vi "GLDL Main.vi"() -> ()   [LabVIEW 2018]
doc: "This template is for the Queued Message Handler design pattern.\n\nThe Event Handling Loop generates messages based on user interface actions.\n\nThe Message Handling Loop processes messages generated by the Event Handling Loop, or by other messages. The messages are string values, so new messages can be added easily to the Message Cases case structure in the Message Handling Loop. Each message cluster can also provide an optional value for Message Data, which is a variant that can be converted to whatever message-specific data is required."
uses:
  controls/GLDL UI Data.ctl
  support/Message Queue/GLDL Message Queue.lvlib
  support/User Event - Stop/GLDL User Event - Stop.lvlib
  support/Message Queue/Enqueue Message (Single).vi
  support/Error Handling/GLDL Error Handling.lvlib
  <vilib>/ErrorRing/Error Ring.xnode
  <vilib>/Utility/error.llb/Error Cluster From Error Code.vi
  support/Message Queue/Message Cluster.ctl
  support/Message Queue/All Message Queues.ctl
  Great Lakes Downloads/support/Message Queue/Enqueue Message (Single).vi
  controls/Connected Indicator.ctl
  controls/Processing Loop State.ctl
  controls/Output Indicator.ctl
  controls/Save Path Control.ctl
  controls/COM Port Control.ctl
  controls/Date Control.ctl
  controls/Disconnect Control.ctl
  controls/Clear Control.ctl
  controls/Exit Control.ctl
  controls/Download Control.ctl
  controls/Station ID Indicator.ctl
  controls/Reboot Control.ctl
  controls/IP Phone Number Control.ctl
panel:
  in  "End Time":T1=timestamp(3579694921.225491 s since 1904-01-01) format="%<%m/%d/%Y %H:%M:%S>T"
  in  "Password":string="akl"
  in  "Username":string="super"
  in  "REBOOT":T2
  out "Station ID":T3
  in  "Start Time":T1=timestamp(3579694921.225491 s since 1904-01-01) format="%<%m/%d/%Y %H:%M:%S>T"
  out "Connected?":T4
  in  "Modem COM Port":T5="COM1"
  in  "Clear Indicator":T6
  in  "IP or Phone Number":T7="9,17578424450"
  in  "Save Path":T8
  out "Output":T9
  in  "Download Data":T10
  in  "Connect to Station":T11
  in  "Exit":T12
  # "9,,,17578424450"
  # "9,14197981041,,,#33,,#33,,#33,,#33"
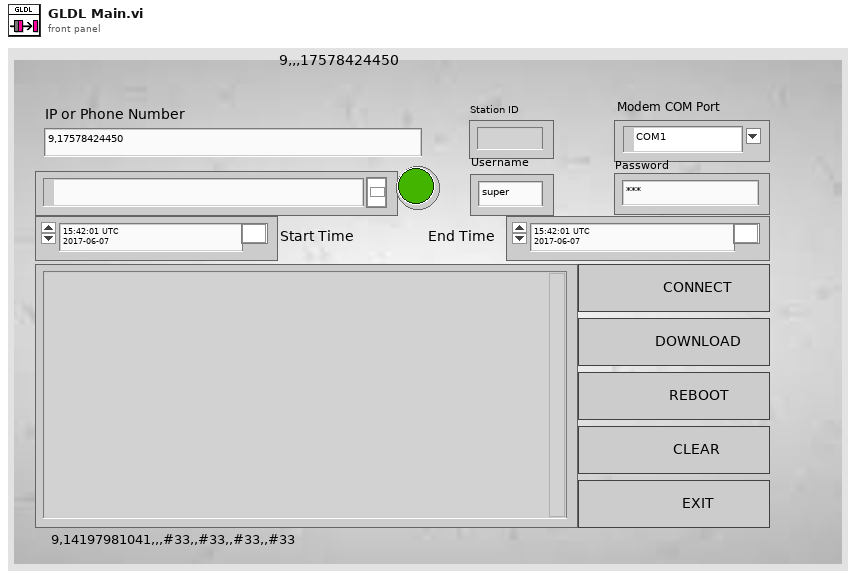
[diagram p1: front panel]
types:
  T1 = typedef "Date Control.ctl" = timestamp
  T2 = typedef "Reboot Control.ctl" = bool
  T3 = typedef "Station ID Indicator.ctl" = string
  T4 = typedef "Connected Indicator.ctl" = bool
  T5 = typedef "COM Port Control.ctl" = refnum<visa-resource-name>
  T6 = typedef "Clear Control.ctl" = bool
  T7 = typedef "IP Phone Number Control.ctl" = string
  T8 = typedef "Save Path Control.ctl" = path
  T9 = typedef "Output Indicator.ctl" = string
  T10 = typedef "Download Control.ctl" = bool
  T11 = typedef "Disconnect Control.ctl" = bool
  T12 = typedef "Exit Control.ctl" = bool
  T13 = typedef "GLDL UI Data.ctl" = cluster{"Data Display":string, "FP Control Refs":cluster{"Connect to Station Ref":refnum<vi>, "Download Ref":refnum<vi>, "Exit Button Ref":refnum<vi>, "Start Date Refnum":refnum<vi>, "End Date Refnum":refnum<vi>, "Path":refnum<vi>, "COM Port":refnum<visa-resource-name>, "IP or Phone Ref":refnum<vi>, "TCPIP ID":refnum<k5>, "Reboot Refnum":refnum<vi>, "Datafile Refnum":refnum<file>}, "FP Indicator Refs":cluster{"Connected Refnum":refnum<vi>, "Data Display Ref":refnum<vi>, "Station ID Ref":refnum<vi>}, "User Events":cluster{"Stop":refnum<user-event>, "Update Display":refnum<user-event>}, "Message Queues":T14, "IS IP?":bool, "Downloading?":bool, "DCP Version":enum16{"XPert", "XPert2"}, "Processing Loop State":T15, "Username":refnum<vi>, "Password":refnum<vi>}
  T14 = typedef "GLDL Message Queue.lvlib/All Message Queues.ctl" = cluster{"UI":refnum<queue>, "ACQUISITION":refnum<queue>, "PROCESSING":refnum<queue>, "LOGGING":refnum<queue>}
  T15 = typedef "Processing Loop State.ctl" = enum16{"Get Station  ID", "Change Directory SD Card", "Change Directory Storage Card", "Downloading", "Idle in DL Directory"}
  T16 = cluster{"Stop":refnum<user-event>, "Update Display":refnum<user-event>}
  T17 = enum16{"Standard", "Buffered", "CRLF", "Immediate"}
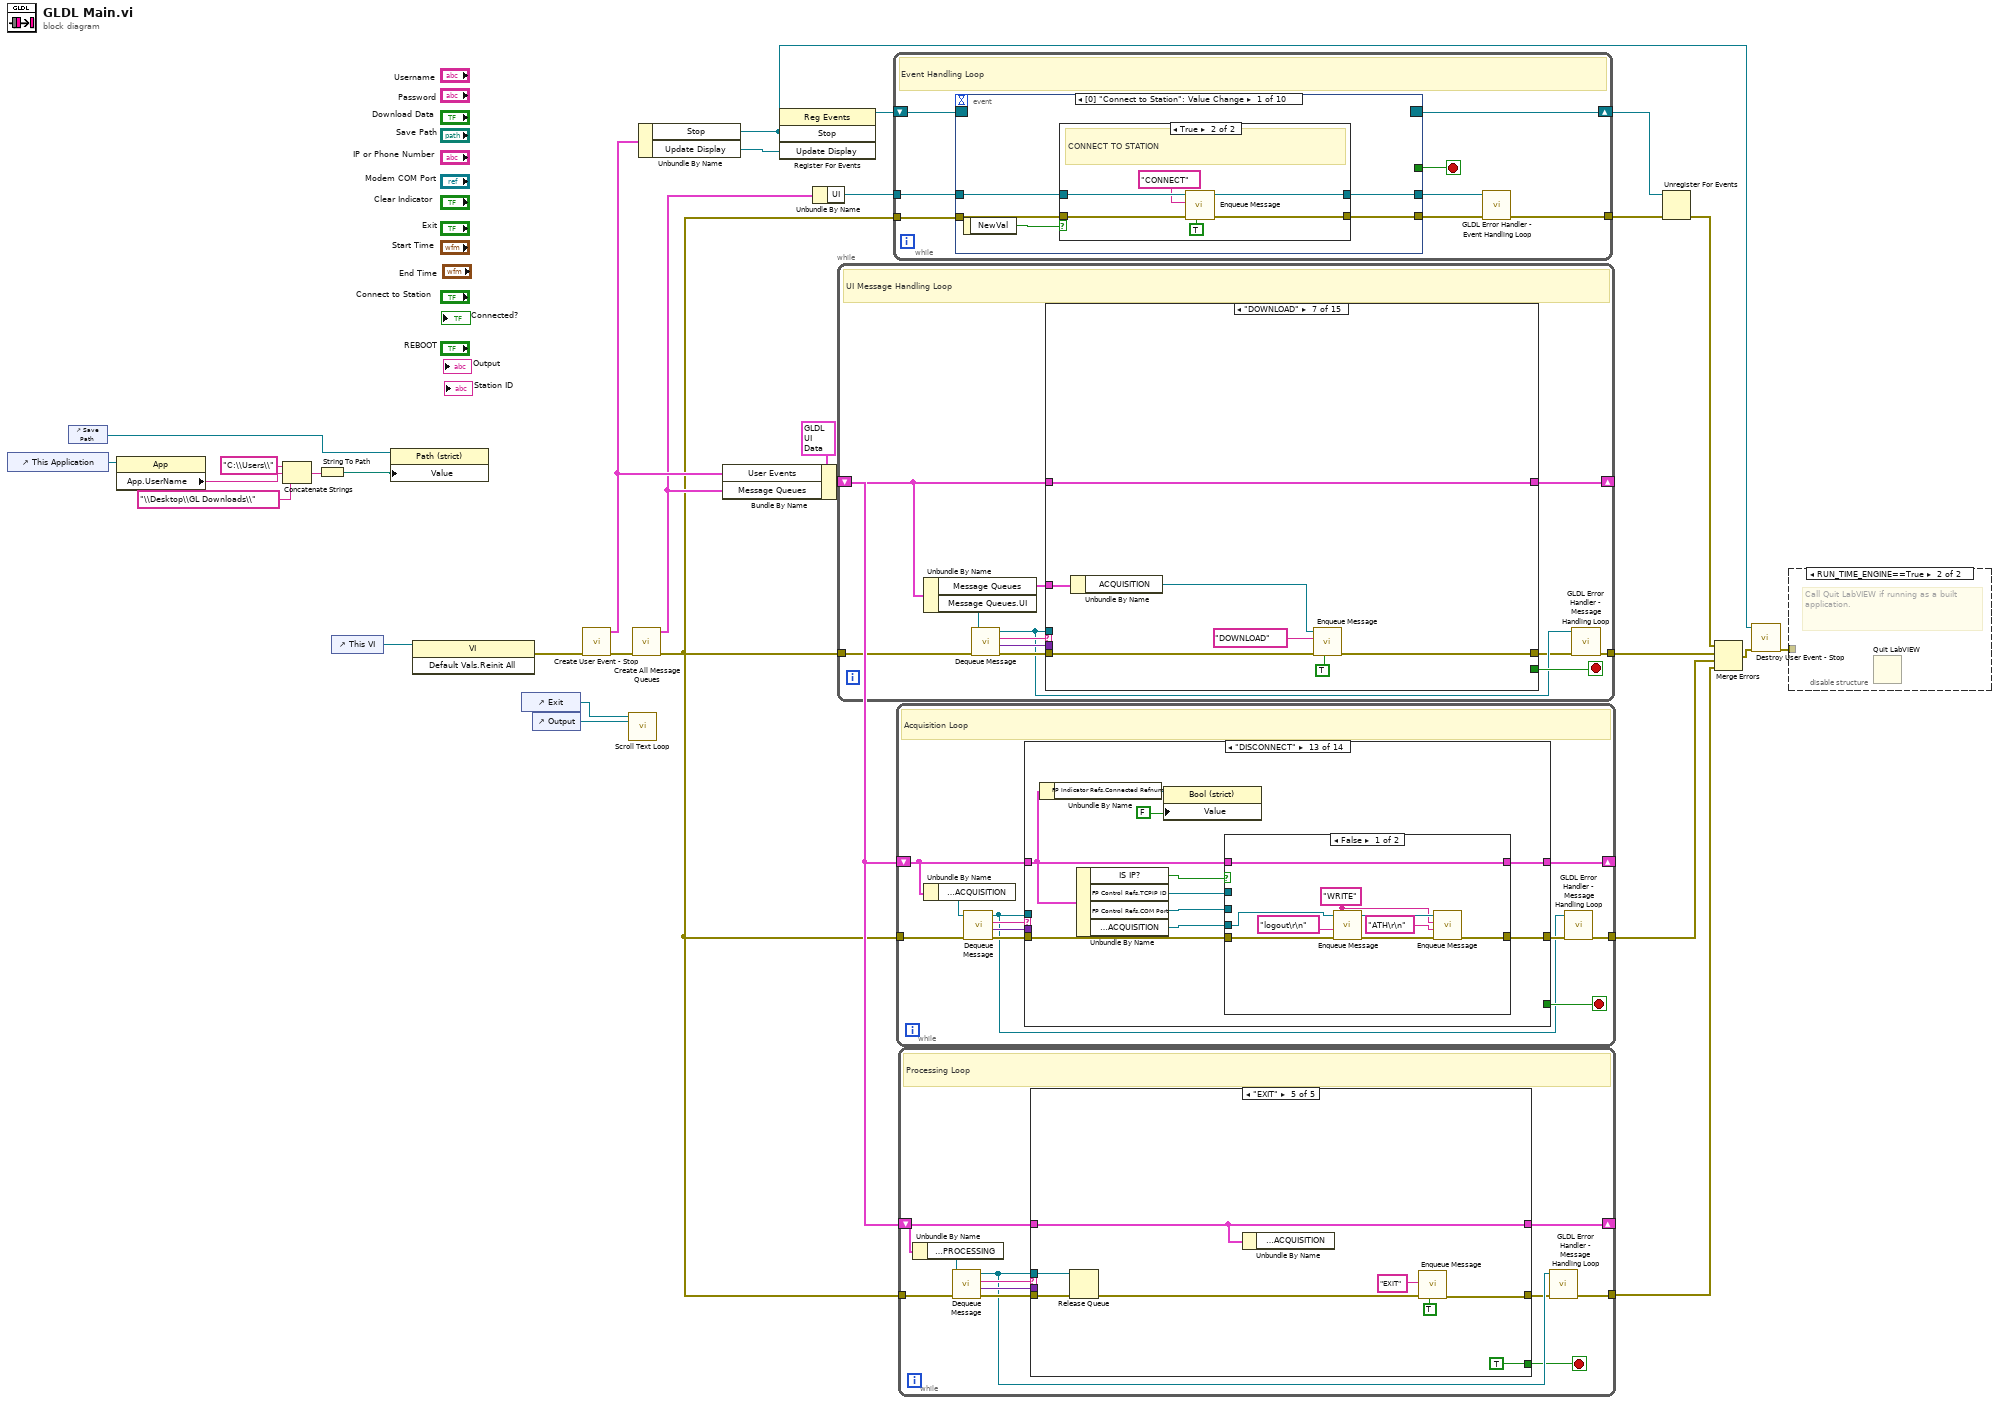
[diagram p0: block diagram]
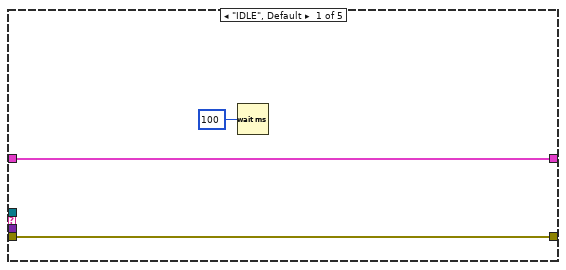
[diagram p2: hidden frame]
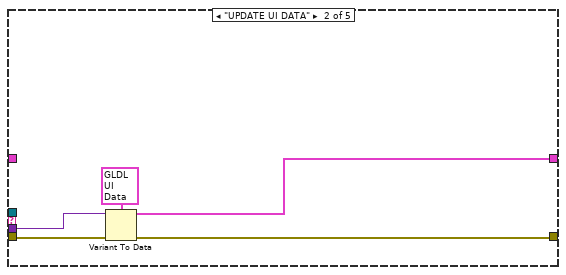
[diagram p3: hidden frame]
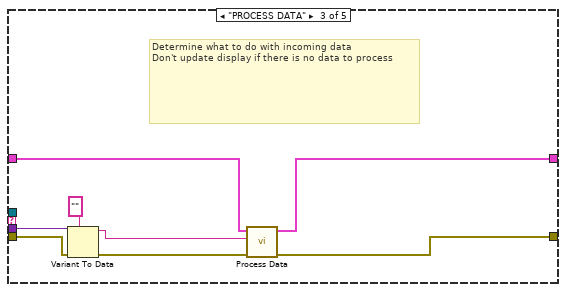
[diagram p4: hidden frame]
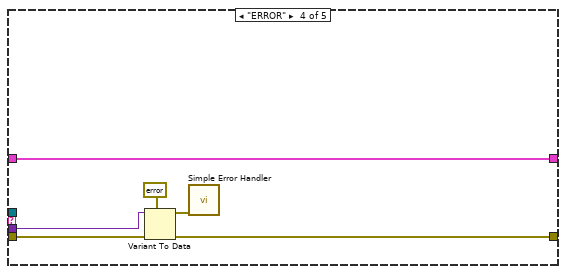
[diagram p5: hidden frame]
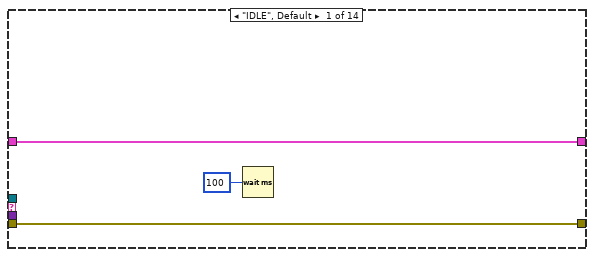
[diagram p6: hidden frame]
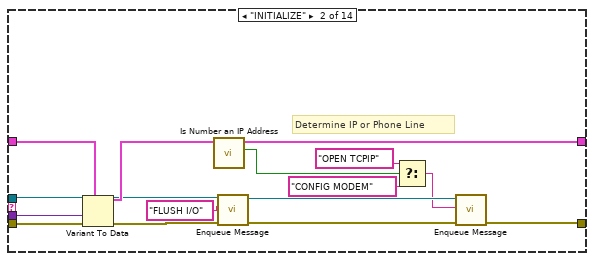
[diagram p7: hidden frame]
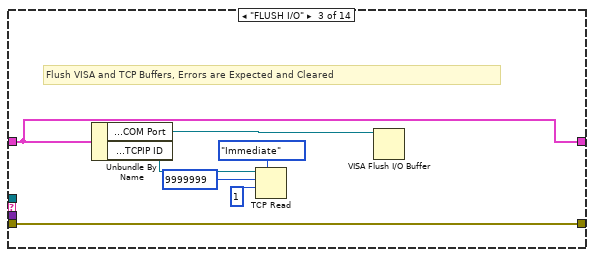
[diagram p8: hidden frame]
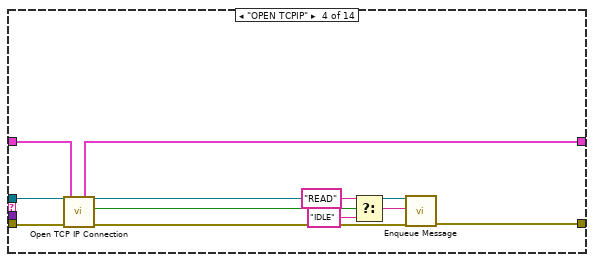
[diagram p9: hidden frame]
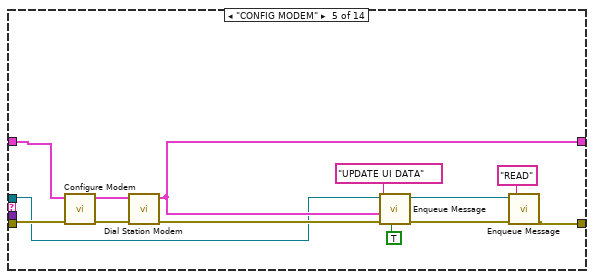
[diagram p10: hidden frame]
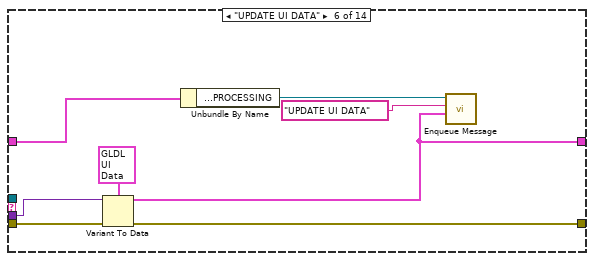
[diagram p11: hidden frame]
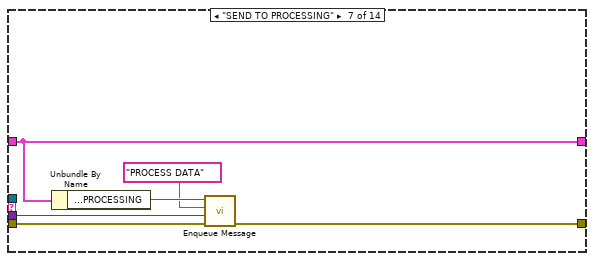
[diagram p12: hidden frame]
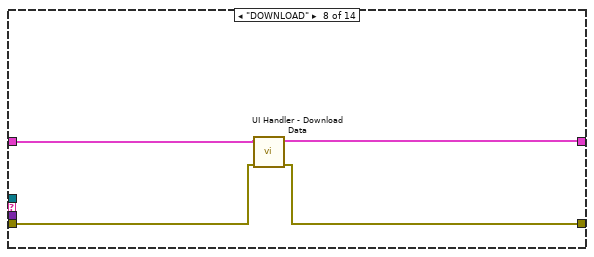
[diagram p13: hidden frame]
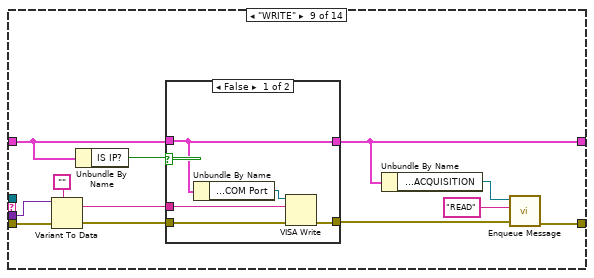
[diagram p14: hidden frame]
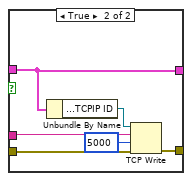
[diagram p15: hidden frame]
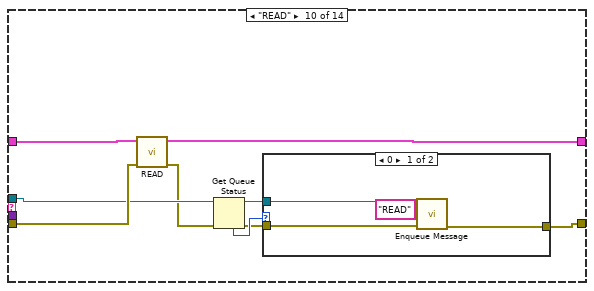
[diagram p16: hidden frame]
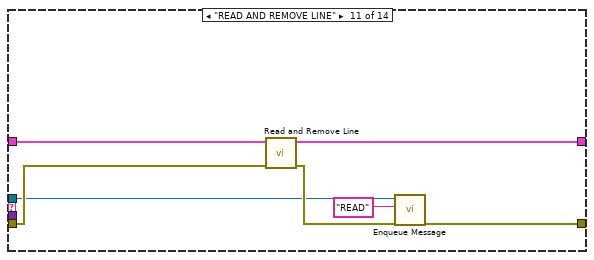
[diagram p18: hidden frame]
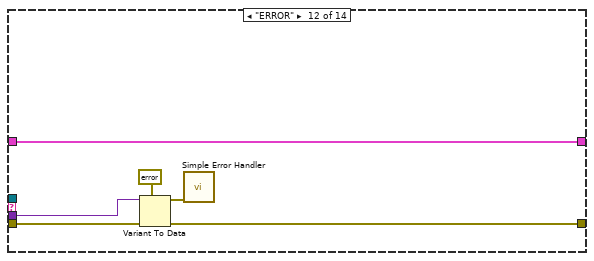
[diagram p19: hidden frame]
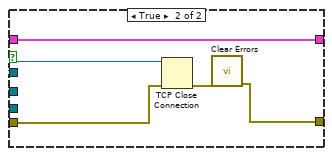
[diagram p20: hidden frame]
diagram:
  n1 = control-ref of="This Application"() -> (w9:refnum<vi>)
  n2 = control-ref of="Save Path"() -> (w3:refnum<vi>)
  n3 = property class="App"(reference=w9) -> ("App.UserName"=w7:string)  [unwired: 1 in, 2 out]
  n4 = Concatenate Strings("C:\\Users\\" ("string"), w7, "\\Desktop\\GL Downloads\\" ("string")) -> (w5:string)
  n5 = String To Path(string=w5) -> (path=w4:path)
  n6 = control-ref of="This VI"() -> (w16:refnum<vi>)
  n7 = property on="Property Node" class="Path (strict)"(reference=w3, "Value"=w4) -> ()  [unwired: 1 in, 2 out]
  n8 = invoke class="VI" method="Default Vals.Reinit All"(reference=w16) -> (error out=w15:errorcluster)  [unwired: 2 in, 2 out]
  n9 = control-ref of="Exit"() -> (w1:refnum<vi>)
  n10 = control-ref of="Output"() -> (w2:refnum<vi>)
  n11 = call "Create User Event - Stop.vi"("error in (no error)"=w15) -> ("error out"=w27:errorcluster, "User Events"=w17:T16)  [unwired: 9 in]
  n12 = call "Scroll Text Loop.vi"("Output Ref"=w2, "Exit Ref"=w1) -> ()  [unwired: 10 in]
  n13 = call "Create All Message Queues.vi"("error in (no error)"=w27) -> ("error out"=w10:errorcluster, "Message Queues out"=w13:T14)  [unwired: 9 in]
  n14 = Unbundle By Name(w17) -> ("Stop"=w20:refnum<user-event>, "Update Display"=w19:refnum<user-event>)
  n15 = Bundle By Name(cluster=T13 {"Data Display"="", "FP Control Refs"={"Connect to Station Ref"=refnum, "Download Ref"=refnum, "Exit Button Ref"=refnum, "Start Date Refnum"=refnum, "End Date Refnum"=refnum, "Path"=refnum, "COM Port"="", "IP or Phone Ref"=refnum, "TCPIP ID"=refnum, "Reboot Refnum"=refnum, "Datafile Refnum"=refnum}, "FP Indicator Refs"={"Connected Refnum"=refnum, "Data Display Ref"=refnum, "Station ID Ref"=refnum}, "User Events"={"Stop"=refnum, "Update Display"=refnum}, "Message Queues"={"UI"=refnum, "ACQUISITION"=refnum, "PROCESSING"=refnum, "LOGGING"=refnum}, "IS IP?"=FALSE, "Downloading?"=FALSE, "DCP Version"=enum."XPert", "Processing Loop State"=enum."Get Station  ID", "Username"=refnum, "Password"=refnum} ("Data Cluster"), "User Events"=w17, "Message Queues"=w13) -> (w11:T13)
  n16 = register-events(w20, w19) -> (reference out=w21:refnum<event-registration>)  [unwired: 2 in, 1 out]
  n17 = Unbundle By Name(w13) -> ("UI"=w28:refnum<queue>)
  n18 = while {
    shift-right: [w41] -> _
    shift-left: w11 -> [w32]
    tunnel: w10 -> [w39]
    tunnel: [w34] -> w29
    stop <- w40 stop-if-true
    # "UI Message Handling Loop"
    n19 = Unbundle By Name(w32) -> ("Message Queues"=w30:T14, "Message Queues.UI"=w31:refnum<queue>)
    n20 = call "Dequeue Message.vi"("error in (no error)"=w39, "Message Queue"=w31) -> ("error out"=w38:errorcluster, "Message Data"=w36:variant, "Message"=w37:string, "dup Message Queue"=w35:refnum<queue>)  [unwired: 6 in]
    n21 = case "Message Cases" shown="\"DOWNLOAD\"" w37 {
      selector: w37 -> [_ _ _ _ _ _ _ _ _ _ _ _ _ _ w157]
      tunnel: w35 -> [w62 _ _ _ _ _ _ _ _ _ _ w139 _ w156 _]
      tunnel: w38 -> [w63 w70 w76 w83 w87 w101 w112 w120 w124 w130 w136 w142 w144 w150 _]
      tunnel: [w51 w69 w74 w82 w92 w105 w111 w118 w123 w130 w131 w140 w144 w154 w158] -> w33
      tunnel: w32 -> [w67 _ w73 w85 w96 w108 w110 w117 w127 w128 w135 w141 w143 w152 w159]
      tunnel: [w48 w68 w73 w84 w96 w108 w110 w116 w127 w129 w135 w141 w143 w152 w159] -> w41
      tunnel: [_ _ _ _ _ _ _ _ _ _ _ _ _ TRUE _] -> w40
      tunnel: w36 -> [_ w71 _ w81 _ _ _ w119 w125 _ w134 _ _ _ _]
      tunnel: w30 -> [w50 _ w78 _ w97 w107 w114 _ _ _ _ _ _ _ _]
      frame "INITIALIZE" {
        w61 = ""  # Initial Message
        n22 = Unbundle By Name(w50) -> ("ACQUISITION"=w49:refnum<queue>)
        n23 = control-ref of="Connected?"() -> (w57:refnum<vi>)
        n24 = control-ref of="Connect to Station"() -> (w65:refnum<vi>)
        n25 = control-ref of="Download Data"() -> (w58:refnum<vi>)
        n26 = control-ref of="Exit"() -> (w64:refnum<vi>)
        n27 = control-ref of="End Time"() -> (w42:refnum<vi>)
        n28 = control-ref of="REBOOT"() -> (w47:refnum<vi>)
        n29 = control-ref of="Start Time"() -> (w43:refnum<vi>)
        n30 = control-ref of="Username"() -> (w45:refnum<vi>)
        n31 = control-ref of="Password"() -> (w44:refnum<vi>)
        n32 = control-ref of="Station ID"() -> (w54:refnum<vi>)
        n33 = control-ref of="IP or Phone Number"() -> (w56:refnum<vi>)
        n34 = control-ref of="Output"() -> (w66:refnum<vi>)
        n35 = call-poly "Enqueue Message.vi"("error in (no error)"=w63, "Message Data"="Initial Message\r\n" ("Initial Message"), "Message"="UPDATE DISPLAY" ("Initial Message"), "Message Queue"=w62) -> ("error out"=w52:errorcluster)  [unwired: 6 in, 1 out]
        n36 = control-ref of="Save Path"() -> (w46:refnum<vi>)
        n37 = property on="Modem COM Port" class="VISAName (strict)"() -> ("Value"=w55:T5)  [unwired: 2 in, 2 out]
        n38 = Bundle By Name(cluster=w67, "Username"=w45, "Password"=w44, "FP Control Refs.Reboot Refnum"=w47, "FP Indicator Refs.Station ID Ref"=w54, "FP Control Refs.IP or Phone Ref"=w56, "FP Indicator Refs.Connected Refnum"=w57, "FP Control Refs.Connect to Station Ref"=w65, "FP Control Refs.Download Ref"=w58, "FP Indicator Refs.Data Display Ref"=w66, "FP Control Refs.Exit Button Ref"=w64, "Data Display"=w61, "FP Control Refs.End Date Refnum"=w42, "FP Control Refs.Start Date Refnum"=w43, "FP Control Refs.COM Port"=w55, "FP Control Refs.Path"=w46) -> (w48:T13)
        n39 = call-poly "Enqueue Message.vi"("error in (no error)"=w52, "Message Data"=w48, "Message"="UPDATE UI DATA" ("Initial Message"), "Message Queue"=w49) -> ("error out"=w51:errorcluster)  [unwired: 6 in, 1 out]
      }
      frame "UPDATE UI DATA" {
        n40 = Variant To Data(error in=w70, type=T13 {"Data Display"="", "FP Control Refs"={"Connect to Station Ref"=refnum, "Download Ref"=refnum, "Exit Button Ref"=refnum, "Start Date Refnum"=refnum, "End Date Refnum"=refnum, "Path"=refnum, "COM Port"="", "IP or Phone Ref"=refnum, "TCPIP ID"=refnum, "Reboot Refnum"=refnum, "Datafile Refnum"=refnum}, "FP Indicator Refs"={"Connected Refnum"=refnum, "Data Display Ref"=refnum, "Station ID Ref"=refnum}, "User Events"={"Stop"=refnum, "Update Display"=refnum}, "Message Queues"={"UI"=refnum, "ACQUISITION"=refnum, "PROCESSING"=refnum, "LOGGING"=refnum}, "IS IP?"=FALSE, "Downloading?"=FALSE, "DCP Version"=enum."XPert", "Processing Loop State"=enum."Get Station  ID", "Username"=refnum, "Password"=refnum} ("Data Cluster"), Variant=w71) -> (data=w68:T13, error out=w69:errorcluster)
      }
      frame "CONNECT" {
        # "Tell the Acquisition Loop to Connect to Station"
        n41 = Unbundle By Name(w78) -> ("ACQUISITION"=w77:refnum<queue>)
        n42 = call-poly "Enqueue Message.vi"("error in (no error)"=w76, "Message Data"=w73, "Message"="INITIALIZE", "Message Queue"=w77) -> ("error out"=w74:errorcluster)  [unwired: 6 in, 1 out]
      }
      frame "COM PORT" {
        n43 = Variant To Data(error in=w83, type=refnum<visa-resource-name> refnum ("FP Control Refs.COM Port"), Variant=w81) -> (data=w79:refnum<visa-resource-name>, error out=w82:errorcluster)
        n44 = Bundle By Name(cluster=w85, "FP Control Refs.COM Port"=w79) -> (w84:T13)
      }
      frame "DISCONNECT" {
        # "Tell the Acquisition Loop to Connect to Station"
        n45 = Unbundle By Name(w97) -> ("ACQUISITION"=w94:refnum<queue>)
        n46 = Flush Queue(queue=w94, error in (no error)=w87) -> (queue out=w93:refnum<queue>, error out=w86:errorcluster)  [unwired: 1 out]
        n47 = call-poly "Enqueue Message.vi"("Priority Message? (F)"=TRUE, "error in (no error)"=w86, "Message Data"=w96, "Message"="DISCONNECT", "Message Queue"=w93) -> ("error out"=w90:errorcluster, "dup Message Queue"=w89:refnum<queue>)  [unwired: 5 in]
        n48 = call-poly "Enqueue Message.vi"("error in (no error)"=w90, "Message"="READ", "Message Queue"=w89) -> ("error out"=w88:errorcluster)  [unwired: 7 in, 1 out]
        n49 = Merge Errors(w88) -> (w92:errorcluster)
      }
      frame "REBOOT" {
        n50 = Unbundle By Name(w107) -> ("ACQUISITION"=w102:refnum<queue>)
        n51 = Flush Queue(queue=w102, error in (no error)=w101) -> (queue out=w99:refnum<queue>, error out=w100:errorcluster)  [unwired: 1 out]
        n52 = call-poly "Enqueue Message.vi"("Priority Message? (F)"=TRUE, "error in (no error)"=w100, "Message Data"="reboot\r\n" ("Message"), "Message"="WRITE", "Message Queue"=w99) -> ("error out"=w105:errorcluster)  [unwired: 5 in, 1 out]
      }
      frame "DOWNLOAD" {
        # "Download specified data from station."
        n53 = Unbundle By Name(w114) -> ("ACQUISITION"=w113:refnum<queue>)
        n54 = call-poly "Enqueue Message.vi"("Priority Message? (F)"=TRUE, "error in (no error)"=w112, "Message"="DOWNLOAD" ("Initial Message"), "Message Queue"=w113) -> ("error out"=w111:errorcluster)  [unwired: 6 in, 1 out]
      }
      frame "UPDATE DISPLAY" {
        # "Update Display - Convert the message data to a string to display in the Data Display indicator."
        n55 = call "GLDL Update Display.vi"("error in (no error)"=w120, "Message Data"=w119, "Data Cluster in"=w117) -> ("error out"=w118:errorcluster, "Data Cluster out"=w116:T13)  [unwired: 7 in]
      }
      frame "UPDATE ID" {
        n56 = Variant To Data(error in=w124, type="", Variant=w125) -> (data=w122:string, error out=w123:errorcluster)
        n57 = Unbundle By Name(w127) -> ("FP Indicator Refs.Station ID Ref"=w126:refnum<vi>)
        n58 = property class="Str (strict)"(reference=w126, "Value"=w122) -> ()  [unwired: 1 in, 2 out]
      }
      frame "CLEAR" {
        n59 = call "GLDL Clear Data Display.vi"("Data Cluster in"=w128) -> ("Data Cluster out"=w129:T13)  [unwired: 10 in]
      }
      frame "ERROR" {
        # "#CodeRecommended - If you ever change the name of this \"Error\" message, you'll need to update the name in the Check Loop Error.vi as well."
        # "#CodeRecommended - Consider creating a system for logging errors in some way. These errors are for notification purposes only. Handling of specific errors should be performed in the message frames that generated the error."
        # "Error - Display an error dialog. This message is sent by the \"Error Handler\" VIs at the end of other loops in this application."
        n60 = Variant To Data(error in=w136, type=errorcluster {"status"=FALSE, "code"=0, "source"=""} ("error constant"), Variant=w134) -> (data=w132:errorcluster, error out=w131:errorcluster)
        n61 = call <vilib>:"Simple Error Handler.vi"("error in (no error)"=w132) -> ()  [unwired: 4 in, 5 out]
      }
      frame "CONFIRM QUIT" {
        # "#CodeNeeded - If you want to provide an \"Are you sure\" dialog (or some other notification) before the application exits, place that code here. This message is typically sent from a Panel Close? event."
        # "Confirm Quit - Message that can confirm whether or not the user wants to exit the application."
        n62 = call-poly "Enqueue Message.vi"("Priority Message? (F)"=TRUE, "error in (no error)"=w142, "Message"="EXIT", "Message Queue"=w139) -> ("error out"=w140:errorcluster)  [unwired: 6 in, 1 out]
      }
      frame "---Copy This Frame---" {
        # "Duplicate this frame when creating new messages.  Change this comment in the duplicated frame to describe this message."
      }
      frame "EXIT" {
        # "Stop the VI"
        # "Exit application. Add any required cleanup code here."
        n63 = Release Queue(queue=w156, error in (no error)=w150) -> (error out=w146:errorcluster)  [unwired: 1 in, 2 out]
        n64 = Unbundle By Name(w152) -> ("User Events.Stop"=w151:refnum<user-event>, "Message Queues.PROCESSING"=w147:refnum<queue>)
        n65 = call-poly "Enqueue Message.vi"("Priority Message? (F)"=TRUE, "error in (no error)"=w146, "Message"="EXIT", "Message Queue"=w147) -> ("error out"=w145:errorcluster)  [unwired: 6 in, 1 out]
        n66 = call "Fire User Event - Stop.vi"("error in (no error)"=w145, "User Event - Stop"=w151) -> ("error out"=w153:errorcluster)  [unwired: 9 in]
        n67 = Merge Errors(w153) -> (w154:errorcluster)
      }
      frame Default {
        # "'Default' case only runs if there is a message that isn't defined in any of the other cases.  Output a programming error."
        n68 = xnode "Error Ring"("parameter 0"=w157) -> ("error out"=w158:errorcluster)
      }
    }
    n69 = call "GLDL Error Handler - Message Handling Loop.vi"("error in (no error)"=w33, "Message Queue"=w35) -> ("dup error in"=w34:errorcluster)  [unwired: 8 in, 1 out]
  }
  n70 = while {
    tunnel: w28 -> [w174]
    shift-right: [w172] -> w24
    shift-left: w21 -> [w173]
    tunnel: [w168] -> w22
    tunnel: w10 -> [w167]
    stop <- w170 stop-if-true
    # "Event Handling Loop"
    n71 = event shown="[0] \"Connect to Station\": Value Change" {
      selector: w173 -> [_ _ _ _ _ _ _ _ _ _]
      dyn-events: [_ _ _ _ _ _ _ _ _ _] -> w172
      timeout: _ -> [_ _ _ _ _ _ _ _ _ _]
      tunnel: [_ _ _ _ _ _ _ _ w231 _] -> w170
      tunnel: w174 -> [w179 w196 w200 w209 w215 w221 w223 w229 w230 w235]
      tunnel: [w177 w194 w201 w206 w212 w220 _ w228 _ _] -> w171
      tunnel: [w178 w195 w199 w208 w214 w219 w223 w227 w230 w233] -> w169
      tunnel: w167 -> [w175 w193 w202 w204 w210 w216 _ w224 _ w232]
      event Value Change {
        n72 = event-data() -> ("NewVal"=w176:T11)  [unwired: 1 in]
        n73 = case shown="True" w176 {
          tunnel: w179 -> [w185 w191]
          tunnel: [w183 w190] -> w178
          tunnel: [w182 w188] -> w177
          tunnel: w175 -> [w181 w187]
          frame False {
            # "DISCONNECT FROM STATION"
            n74 = call-poly "Enqueue Message.vi"("Priority Message? (F)"=TRUE, "error in (no error)"=w181, "Message"="DISCONNECT", "Message Queue"=w185) -> ("error out"=w182:errorcluster, "dup Message Queue"=w183:refnum<queue>)  [unwired: 6 in]
          }
          frame True {
            # "CONNECT TO STATION"
            n75 = call-poly "Enqueue Message.vi"("Priority Message? (F)"=TRUE, "error in (no error)"=w187, "Message"="CONNECT", "Message Queue"=w191) -> ("error out"=w188:errorcluster, "dup Message Queue"=w190:refnum<queue>)  [unwired: 6 in]
          }
        }
      }
      event Value Change {
        n76 = event-data() -> ("NewVal"=w192:T5)  [unwired: 1 in]
        n77 = call-poly "Enqueue Message.vi"("error in (no error)"=w193, "Message Data"=w192, "Message"="COM PORT", "Message Queue"=w196) -> ("error out"=w194:errorcluster, "dup Message Queue"=w195:refnum<queue>)  [unwired: 6 in]
      }
      event Value Change {
        n78 = event-data() -> ()  [unwired: 1 in, 1 out]
        n79 = call-poly "Enqueue Message.vi"("error in (no error)"=w202, "Message"="REBOOT", "Message Queue"=w200) -> ("error out"=w201:errorcluster, "dup Message Queue"=w199:refnum<queue>)  [unwired: 7 in]
      }
      event Value Change {
        n80 = event-data() -> ()  [unwired: 1 in, 1 out]
        n81 = property on="Download Data" class="Bool (strict)"(error in=w204, "Value"=FALSE) -> (error out=w203:errorcluster)  [unwired: 1 in, 1 out]
        n82 = call-poly "Enqueue Message.vi"("error in (no error)"=w203, "Message"="DOWNLOAD", "Message Queue"=w209) -> ("error out"=w206:errorcluster, "dup Message Queue"=w208:refnum<queue>)  [unwired: 7 in]
      }
      event Value Change {
        n83 = event-data() -> ("OldVal"=w211:T6)  [unwired: 1 in]
        n84 = property on="Clear Indicator" class="Bool (strict)"("Value"=w211) -> ()  [unwired: 2 in, 2 out]
        n85 = call-poly "Enqueue Message.vi"("error in (no error)"=w210, "Message"="CLEAR", "Message Queue"=w215) -> ("error out"=w212:errorcluster, "dup Message Queue"=w214:refnum<queue>)  [unwired: 7 in]
      }
      event Panel Close? {
        n86 = event-data() -> ()  [unwired: 1 in, 1 out]
        n87 = call-poly "Enqueue Message.vi"("Priority Message? (F)"=TRUE, "error in (no error)"=w216, "Message"="Confirm Quit", "Message Queue"=w221) -> ("error out"=w220:errorcluster, "dup Message Queue"=w219:refnum<queue>)  [unwired: 6 in]
        n88 = event-data("Discard?"=TRUE) -> ()  [unwired: 1 in, 1 out]
      }
      event Application Instance Close {
        # "#CodeRecommended - However, any code placed in this event frame is guaranteed to run to completion, so add any cleanup code that absolutely must happen here."
        n89 = event-data() -> ()  [unwired: 1 in, 1 out]
      }
      event Value Change {
        n90 = event-data() -> ()  [unwired: 1 in, 1 out]
        n91 = call-poly "Enqueue Message.vi"("Priority Message? (F)"=TRUE, "error in (no error)"=w224, "Message"="EXIT", "Message Queue"=w229) -> ("error out"=w228:errorcluster, "dup Message Queue"=w227:refnum<queue>)  [unwired: 6 in]
      }
      event User Event {
        w231 = TRUE ("Discard?")
        n92 = event-data() -> ()  [unwired: 1 in, 1 out]
        n93 = local write "Exit"(w231) -> ()
      }
      event User Event {
        n94 = event-data() -> ("Update Display Event"=w234:string)  [unwired: 1 in]
        n95 = call-poly "Enqueue Message.vi"("error in (no error)"=w232, "Message Data"=w234, "Message"="UPDATE DISPLAY" ("Initial Message"), "Message Queue"=w235) -> ("dup Message Queue"=w233:refnum<queue>)  [unwired: 6 in, 1 out]
      }
    }
    n96 = call "GLDL Error Handler - Event Handling Loop.vi"("error in (no error)"=w171, "Message Queue"=w169) -> ("dup error in"=w168:errorcluster)  [unwired: 8 in, 1 out]
  }
  n97 = while {
    tunnel: [w247] -> w14
    tunnel: w10 -> [w245]
    shift-right: [w239] -> _
    shift-left: w11 -> [w238]
    stop <- w240 stop-if-true
    # "Acquisition Loop"
    n98 = Unbundle By Name(w238) -> ("Message Queues.ACQUISITION"=w246:refnum<queue>)
    n99 = call "Dequeue Message.vi"("error in (no error)"=w245, "Message Queue"=w246) -> ("error out"=w244:errorcluster, "Message Data"=w243:variant, "Message"=w242:string, "dup Message Queue"=w237:refnum<queue>)  [unwired: 6 in]
    n100 = case shown="\"DISCONNECT\"" w242 {
      tunnel: w244 -> [w250 w262 w266 w276 w287 w302 w307 w313 w323 w345 w355 w360 w366 w392]
      tunnel: w243 -> [_ w259 _ _ _ w301 w305 _ w321 _ _ w358 _ _]
      tunnel: w237 -> [_ w261 _ w273 w284 _ _ _ _ w341 w352 _ _ w391]
      tunnel: [w250 w254 w266 w277 w288 w300 w306 w310 w314 w338 w356 w359 w365 w389] -> w241
      tunnel: [_ _ _ _ _ _ _ _ _ _ _ _ _ TRUE] -> w240
      tunnel: [w249 w258 w267 w274 w285 w297 w309 w311 w318 w343 w353 w357 w367 w387] -> w239
      tunnel: w238 -> [w249 w260 w267 w275 w286 w299 w309 w312 w324 w344 w354 w357 w364 w388]
      frame "IDLE", Default {
        n101 = Wait (ms)(milliseconds to wait=u32 100) -> ()  [unwired: 1 out]
      }
      frame "INITIALIZE" {
        # "Determine IP or Phone Line"
        n102 = Variant To Data(error in=w262, type=w260, Variant=w259) -> (data=w263:T13, error out=w264:errorcluster)
        n103 = call "Is Number an IP Address.vi"("UI Data in"=w263) -> ("IS IP?"=w257:bool, "UI Data out"=w258:T13)  [unwired: 9 in]
        n104 = call-poly "Enqueue Message.vi"("error in (no error)"=w264, "Message"="FLUSH I/O", "Message Queue"=w261) -> ("error out"=w253:errorcluster, "dup Message Queue"=w252:refnum<queue>)  [unwired: 7 in]
        n105 = Select(t="OPEN TCPIP" ("Message"), s=w257, f="CONFIG MODEM" ("Message")) -> (s? t:f=w251:string)
        n106 = call-poly "Enqueue Message.vi"("error in (no error)"=w253, "Message"=w251, "Message Queue"=w252) -> ("error out"=w254:errorcluster)  [unwired: 7 in, 1 out]
      }
      frame "FLUSH I/O" {
        # "Flush VISA and TCP Buffers, Errors are Expected and Cleared"
        n107 = Unbundle By Name(w267) -> ("FP Control Refs.COM Port"=w272:refnum<visa-resource-name>, "FP Control Refs.TCPIP ID"=w270:refnum<k5>)
        n108 = TCP Read(connection ID=w270, bytes to read=9999999, 7:T17."Immediate" ("mode (standard)"), 9:1 ("bytes to read")) -> ()  [unwired: 1 in, 3 out]
        n109 = VISA Flush I/O Buffer(VISA resource name=w272) -> ()  [unwired: 2 in, 2 out]
      }
      frame "OPEN TCPIP" {
        n110 = call "Open TCP IP Connection.vi"("error in (no error)"=w276, "Data Cluster in"=w275) -> ("error out"=w282:errorcluster, "Connected?"=w278:bool, "Data Cluster out"=w274:T13)  [unwired: 7 in]
        n111 = Select(t="READ" ("Initial Message"), s=w278, f="IDLE" ("Initial Message")) -> (s? t:f=w280:string)
        n112 = call-poly "Enqueue Message.vi"("error in (no error)"=w282, "Message"=w280, "Message Queue"=w273) -> ("error out"=w277:errorcluster)  [unwired: 7 in, 1 out]
      }
      frame "CONFIG MODEM" {
        n113 = call "Configure Modem.vi"("error in (no error)"=w287, "Data Cluster"=w286) -> ("error out"=w290:errorcluster, "Data Cluster out"=w289:T13)  [unwired: 8 in]
        n114 = call "Dial Station Modem.vi"("error in (no error)"=w290, "Data Cluster in"=w289) -> ("error out (no error)"=w291:errorcluster, "Data Cluster out"=w285:T13)  [unwired: 8 in]
        n115 = call-poly "Enqueue Message.vi"("Priority Message? (F)"=TRUE, "error in (no error)"=w291, "Message Data"=w285, "Message"="UPDATE UI DATA", "Message Queue"=w284) -> ("error out"=w293:errorcluster, "dup Message Queue"=w294:refnum<queue>)  [unwired: 5 in]
        n116 = call-poly "Enqueue Message.vi"("error in (no error)"=w293, "Message"="READ", "Message Queue"=w294) -> ("error out"=w288:errorcluster)  [unwired: 7 in, 1 out]
      }
      frame "UPDATE UI DATA" {
        n117 = Variant To Data(error in=w302, type=T13 {"Data Display"="", "FP Control Refs"={"Connect to Station Ref"=refnum, "Download Ref"=refnum, "Exit Button Ref"=refnum, "Start Date Refnum"=refnum, "End Date Refnum"=refnum, "Path"=refnum, "COM Port"="", "IP or Phone Ref"=refnum, "TCPIP ID"=refnum, "Reboot Refnum"=refnum, "Datafile Refnum"=refnum}, "FP Indicator Refs"={"Connected Refnum"=refnum, "Data Display Ref"=refnum, "Station ID Ref"=refnum}, "User Events"={"Stop"=refnum, "Update Display"=refnum}, "Message Queues"={"UI"=refnum, "ACQUISITION"=refnum, "PROCESSING"=refnum, "LOGGING"=refnum}, "IS IP?"=FALSE, "Downloading?"=FALSE, "DCP Version"=enum."XPert", "Processing Loop State"=enum."Get Station  ID", "Username"=refnum, "Password"=refnum} ("Data Cluster"), Variant=w301) -> (data=w297:T13, error out=w300:errorcluster)
        n118 = Unbundle By Name(w299) -> ("Message Queues.PROCESSING"=w298:refnum<queue>)
        n119 = call-poly "Enqueue Message.vi"("Message Data"=w297, "Message"="UPDATE UI DATA" ("Initial Message"), "Message Queue"=w298) -> ()  [unwired: 7 in, 2 out]
      }
      frame "SEND TO PROCESSING" {
        n120 = Unbundle By Name(w309) -> ("Message Queues.PROCESSING"=w308:refnum<queue>)
        n121 = call-poly "Enqueue Message.vi"("error in (no error)"=w307, "Message Data"=w305, "Message"="PROCESS DATA", "Message Queue"=w308) -> ("error out"=w306:errorcluster)  [unwired: 6 in, 1 out]
      }
      frame "DOWNLOAD" {
        n122 = call "UI Handler - Download Data.vi"("error in (no error)"=w313, "Data Cluster"=w312) -> ("error out"=w310:errorcluster, "Data Cluster out"=w311:T13)  [unwired: 8 in]
      }
      frame "WRITE" {
        n123 = Variant To Data(error in=w323, type="", Variant=w321) -> (data=w319:string, error out=w322:errorcluster)
        n124 = Unbundle By Name(w324) -> ("IS IP?"=w325:bool)
        n125 = case shown="False" w325 {
          tunnel: w324 -> [w327 w334]
          tunnel: w322 -> [w330 w336]
          tunnel: [w329 w335] -> w315
          tunnel: [w327 w334] -> w318
          tunnel: w319 -> [w326 w332]
          frame False {
            n126 = Unbundle By Name(w327) -> ("FP Control Refs.COM Port"=w328:refnum<visa-resource-name>)
            n127 = VISA Write(VISA resource name=w328, write buffer=w326, error in (no error)=w330) -> (error out=w329:errorcluster)  [unwired: 2 out]
          }
          frame True {
            n128 = Unbundle By Name(w334) -> ("FP Control Refs.TCPIP ID"=w333:refnum<k5>)
            n129 = TCP Write(connection ID=w333, data in=w332, error in (no error)=w336, 9:5000 ("timeout ms (25000)")) -> (error out=w335:errorcluster)  [unwired: 2 out]
          }
        }
        n130 = Unbundle By Name(w318) -> ("Message Queues.ACQUISITION"=w316:refnum<queue>)
        n131 = call-poly "Enqueue Message.vi"("error in (no error)"=w315, "Message"="READ" ("Initial Message"), "Message Queue"=w316) -> ("error out"=w314:errorcluster)  [unwired: 7 in, 1 out]
      }
      frame "READ" {
        n132 = call "READ.vi"("error in (no error)"=w345, "Data Cluster in"=w344) -> ("error out"=w340:errorcluster, "Data Cluster out"=w343:T13)  [unwired: 8 in]
        n133 = Get Queue Status(queue=w341, error in (no error)=w340) -> (queue out=w337:refnum<queue>, error out=w339:errorcluster, # elements in queue=w342:i32)  [unwired: 1 in, 5 out]
        n134 = case shown="0" w342 {
          tunnel: w339 -> [w348 w350]
          tunnel: [w349 w350] -> w338
          tunnel: w337 -> [w346 _]
          frame 0 {
            n135 = call-poly "Enqueue Message.vi"("error in (no error)"=w348, "Message"="READ", "Message Queue"=w346) -> ("error out"=w349:errorcluster)  [unwired: 7 in, 1 out]
          }
          frame 21, Default {
          }
        }
      }
      frame "READ AND REMOVE LINE" {
        n136 = call "Read and Remove Line.vi"("error in (no error)"=w355, "Data Cluster in"=w354) -> ("error out"=w356:errorcluster, "Data Cluster out"=w353:T13)  [unwired: 7 in, 1 out]
        n137 = call-poly "Enqueue Message.vi"("Message"="READ", "Message Queue"=w352) -> ()  [unwired: 8 in, 2 out]
      }
      frame "ERROR" {
        n138 = Variant To Data(error in=w360, type=errorcluster {"status"=FALSE, "code"=0, "source"=""} ("error constant"), Variant=w358) -> (data=w362:errorcluster, error out=w359:errorcluster)
        n139 = call <vilib>:"Simple Error Handler.vi"("error in (no error)"=w362) -> ()  [unwired: 4 in, 5 out]
      }
      frame "DISCONNECT" {
        n140 = Unbundle By Name(w364) -> ("FP Indicator Refs.Connected Refnum"=w371:refnum<vi>)
        n141 = Unbundle By Name(w364) -> ("IS IP?"=w368:bool, "FP Control Refs.TCPIP ID"=w369:refnum<k5>, "FP Control Refs.COM Port"=w370:refnum<visa-resource-name>, "Message Queues.ACQUISITION"=w363:refnum<queue>)
        n142 = property class="Bool (strict)"(reference=w371, "Value"=T4 FALSE) -> ()  [unwired: 1 in, 2 out]
        n143 = case shown="False" w368 {
          tunnel: w369 -> [_ w386]
          tunnel: w366 -> [w378 w385]
          tunnel: [w374 w382] -> w365
          tunnel: w370 -> [_ _]
          tunnel: w364 -> [w381 w384]
          tunnel: [w381 w384] -> w367
          tunnel: w363 -> [w380 _]
          frame False {
            w373 = "WRITE" ("write buffer")
            n144 = call-poly "Enqueue Message.vi"("error in (no error)"=w378, "Message Data"="logout\r\n" ("write buffer"), "Message"=w373, "Message Queue"=w380) -> ("error out"=w376:errorcluster, "dup Message Queue"=w377:refnum<queue>)  [unwired: 6 in]
            n145 = call-poly "Enqueue Message.vi"("error in (no error)"=w376, "Message Data"="ATH\r\n" ("write buffer"), "Message"=w373, "Message Queue"=w377) -> ("error out"=w374:errorcluster)  [unwired: 6 in, 1 out]
          }
          frame True {
            n146 = TCP Close Connection(connection ID=w386, error in (no error)=w385) -> (error out=w383:errorcluster)  [unwired: 1 in, 1 out]
            n147 = call <vilib>:"Clear Errors.vi"("error in (no error)"=w383) -> ("error out"=w382:errorcluster)  [unwired: 5 in, 1 out]
          }
        }
      }
      frame "EXIT" {
        n148 = Release Queue(queue=w391, error in (no error)=w392) -> (error out=w390:errorcluster)  [unwired: 1 in, 2 out]
        n149 = call "Exit Acq Loop.vi"("error in (no error)"=w390, "Data Cluster in"=w388) -> ("error out"=w389:errorcluster, "Data Cluster out"=w387:T13)  [unwired: 8 in]
      }
    }
    n150 = call "GLDL Error Handler - Message Handling Loop.vi"("error in (no error)"=w241, "Message Queue"=w237) -> ("dup error in"=w247:errorcluster)  [unwired: 8 in, 1 out]
  }
  n151 = while {
    tunnel: [w404] -> w12
    tunnel: w10 -> [w402]
    shift-right: [w397] -> _
    shift-left: w11 -> [w396]
    stop <- w394 stop-if-true
    # "Processing Loop"
    n152 = Unbundle By Name(w396) -> ("Message Queues.PROCESSING"=w403:refnum<queue>)
    n153 = call "Dequeue Message.vi"("error in (no error)"=w402, "Message Queue"=w403) -> ("error out"=w400:errorcluster, "Message Data"=w399:variant, "Message"=w401:string, "dup Message Queue"=w398:refnum<queue>)  [unwired: 6 in]
    n154 = case shown="\"EXIT\"" w401 {
      tunnel: w398 -> [_ _ _ _ w432]
      tunnel: w400 -> [w405 w411 w419 w423 w433]
      tunnel: w399 -> [_ w409 w420 w421 _]
      tunnel: [w407 w408 w414 w426 w428] -> w397
      tunnel: w396 -> [w407 _ w415 w426 w428]
      tunnel: [w405 w410 w416 w422 w429] -> w395
      tunnel: [_ _ _ _ TRUE] -> w394
      frame "IDLE", Default {
        n155 = Wait (ms)(milliseconds to wait=u32 100) -> ()  [unwired: 1 out]
      }
      frame "UPDATE UI DATA" {
        n156 = Variant To Data(error in=w411, type=T13 {"Data Display"="", "FP Control Refs"={"Connect to Station Ref"=refnum, "Download Ref"=refnum, "Exit Button Ref"=refnum, "Start Date Refnum"=refnum, "End Date Refnum"=refnum, "Path"=refnum, "COM Port"="", "IP or Phone Ref"=refnum, "TCPIP ID"=refnum, "Reboot Refnum"=refnum, "Datafile Refnum"=refnum}, "FP Indicator Refs"={"Connected Refnum"=refnum, "Data Display Ref"=refnum, "Station ID Ref"=refnum}, "User Events"={"Stop"=refnum, "Update Display"=refnum}, "Message Queues"={"UI"=refnum, "ACQUISITION"=refnum, "PROCESSING"=refnum, "LOGGING"=refnum}, "IS IP?"=FALSE, "Downloading?"=FALSE, "DCP Version"=enum."XPert", "Processing Loop State"=enum."Get Station  ID", "Username"=refnum, "Password"=refnum} ("Data Cluster"), Variant=w409) -> (data=w408:T13, error out=w410:errorcluster)
      }
      frame "PROCESS DATA" {
        # "Determine what to do with incoming data\nDon't update display if there is no data to process"
        n157 = Variant To Data(error in=w419, type="" ("data out"), Variant=w420) -> (data=w417:string, error out=w418:errorcluster)
        n158 = call "Process Data.vi"("error in (no error)"=w418, "Data In"=w417, "Data Cluster in"=w415) -> ("error out"=w416:errorcluster, "Data Cluster out"=w414:T13)  [unwired: 7 in]
      }
      frame "ERROR" {
        n159 = Variant To Data(error in=w423, type=errorcluster {"status"=FALSE, "code"=0, "source"=""} ("error constant"), Variant=w421) -> (data=w424:errorcluster, error out=w422:errorcluster)
        n160 = call <vilib>:"Simple Error Handler.vi"("error in (no error)"=w424) -> ()  [unwired: 4 in, 5 out]
      }
      frame "EXIT" {
        n161 = Release Queue(queue=w432, error in (no error)=w433) -> (error out=w427:errorcluster)  [unwired: 1 in, 2 out]
        n162 = Unbundle By Name(w428) -> ()  [unwired: 1 out]
        n163 = call-poly "Enqueue Message.vi"("Priority Message? (F)"=TRUE, "error in (no error)"=w427, "Message"="EXIT") -> ("error out"=w429:errorcluster)  [unwired: 7 in, 1 out]
      }
    }
    n164 = call "GLDL Error Handler - Message Handling Loop.vi"("error in (no error)"=w395, "Message Queue"=w398) -> ("dup error in"=w404:errorcluster)  [unwired: 8 in, 1 out]
  }
  n165 = Unregister For Events(event registration refnum=w24, error in=w22) -> (error out=w25:errorcluster)
  n166 = Merge Errors(w25, w29, w14, w12) -> (w26:errorcluster)
  n167 = call "Destroy User Event - Stop.vi"("error in (no error)"=w26, "User Event - Stop"=w20) -> ("error out"=w23:errorcluster)  [unwired: 9 in]
  n168 = disable-structure shown="RUN_TIME_ENGINE==True" {
    disable-tunnel: w23 -> [_ _]
    frame condition #0 (active) {
    }
    frame condition #1 {
      # "Call Quit LabVIEW if running as a built application."
      n169 = Quit LabVIEW() -> ()  [unwired: 1 in]
    }
  }
